vi "Cartesian Point 2 Array.vi"(2 "Cart Disp":T1) -> (1 "Array":dbl[](array[numeric]))   [LabVIEW 2013]
uses:
  Metadata/Cartesian Point.ctl
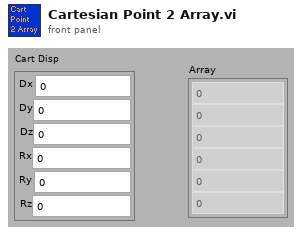
[diagram p1: front panel]
types:
  T1 = typedef "Cartesian Point.ctl" = cluster{"Dx":dbl, "Dy":dbl, "Dz":dbl, "Rx":dbl, "Ry":dbl, "Rz":dbl}
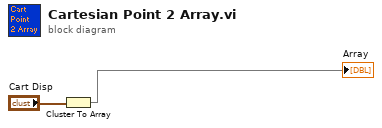
[diagram p0: block diagram]
diagram:
  n1 = Cluster To Array(cluster="Cart Disp") -> (array=→"Array":dbl[])
